vi "action - GitRepo Force Sync to Latest.vi"(8 "error in (no error)":errorcluster, 11 "Path":path) -> (3 "f":string)   [LabVIEW 2017]
doc: "s"
uses:
  <vilib>/Hampel Software Engineering/Git API/Git API/GIT-api.lvclass/GIT-api.ctl
  <vilib>/Hampel Software Engineering/Git API/Git API/Accessors/GIT-Set Working Dir.vi
  <vilib>/Hampel Software Engineering/Git API/Git API/GIT-api.lvclass
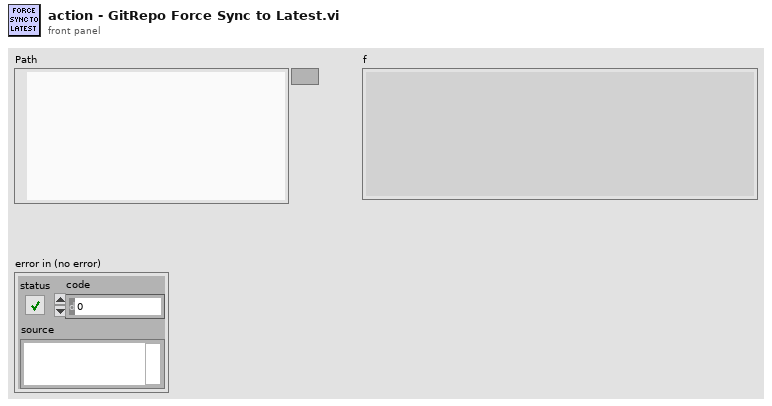
[diagram p1: front panel]
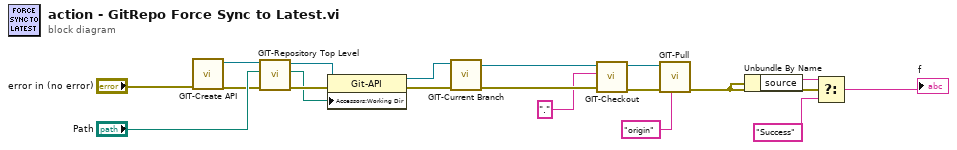
[diagram p0: block diagram]
diagram:
  n1 = call <vilib>:"GIT-Create API.vi"("error in"="error in (no error)") -> ("error out"=w14:errorcluster, "git-api out"=w16:refnum<class "GIT-api.lvclass">)  [unwired: 9 in]
  n2 = call <vilib>:"GIT-Repository Top Level.vi"("error in"=w14, "Current Path"="Path", "git-api in"=w16) -> ("error out"=w19:errorcluster, "Repo Top Level Path"=w17:path, "git-api out"=w18:refnum<class "GIT-api.lvclass">)  [unwired: 6 in]
  n3 = property class="Git-API"(reference=w18, error in=w19, "Accessors:Working Dir"=w17) -> (reference out=w10:refnum<class "GIT-api.lvclass">, error out=w11:errorcluster)
  n4 = call <vilib>:"GIT-Current Branch.vi"("error in"=w11, "git-api in"=w10) -> ("error out"=w9:errorcluster, "git-api out"=w8:refnum<class "GIT-api.lvclass">)  [unwired: 7 in, 1 out]
  n5 = call <vilib>:"GIT-Checkout.vi"("error in"=w9, "branch name"=".", "git-api in"=w8) -> ("error out"=w5:errorcluster, "git-api out"=w6:refnum<class "GIT-api.lvclass">)  [unwired: 7 in]
  n6 = call <vilib>:"GIT-Pull.vi"("param"="origin", "error in"=w5, "git-api in"=w6) -> ("error out"=w2:errorcluster)  [unwired: 7 in, 1 out]
  n7 = Unbundle By Name(w2) -> ("source"=w3:string)
  n8 = Select(t=w3, s=w2, f="Success") -> (s? t:f=→"f":string)
